vi "WriteToFilesMap.vi"(8 "error in (no error)":errorcluster, 11 "Items To Serialize":T1[](array[typedef])) -> (0 "error out":errorcluster)   [LabVIEW 2017]
uses:
  JsonConverters/ApplicationItems.ctl
  JsonConverters/SourceJsonPaths.ctl
  FilesAndOutputPathMap.vi
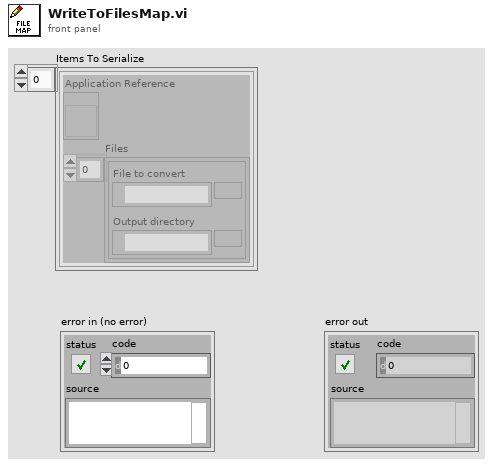
[diagram p1: front panel]
types:
  T1 = typedef "ApplicationItems.ctl" = cluster{"Application Reference":refnum<vi>, "Files":T2[]}
  T2 = typedef "SourceJsonPaths.ctl" = cluster{"File to convert":path, "Output directory":path}
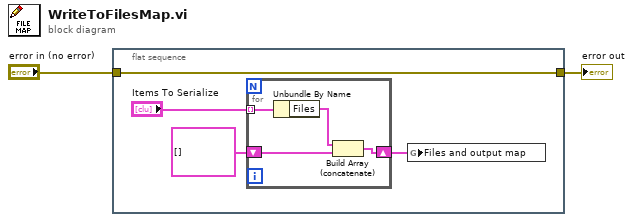
[diagram p0: block diagram]
diagram:
  n1 = flat-sequence {
    tunnel: [w3] -> w2
    tunnel: "error in (no error)" -> [w3]
    frame #0 {
      n2 = for {
        tunnel: "Items To Serialize" -> [w10] mode=indexing
        shift-right: [w7] -> w5
        shift-left: T2[] [] -> [w8]
        n3 = Unbundle By Name(w10) -> ("Files"=w9:T2[])
        n4 = Build Array (concatenate)(w9, w8) -> (w7:T2[])
      }
      n5 = global write "FilesAndOutputPathMap.vi" "Files and output map"(w5) -> ()
    }
  }
  "error out" <- w2
